vi "Simple TCP - Client.vi"() -> ()   [LabVIEW 2020]
doc: "Demonstrates how to open a connection to an TCP server, read the data being sent, and display the data on a chart. This VI is designed to stop if the TCP connection is terminated."
panel:
  out "data out":string
  in  "Server Closed":string="The server VI closed the connection."
  # "Overview: Demonstrates the use of the TCP functions to connect to a TCP server VI and receive data.\nInstructions:\n1. Ensure Simple TCP - Server.vi is already running.\n2. Run the VI.\n3. Click Stop to stop the VI. Note that if you stop the server VI, this VI will stop automatically."
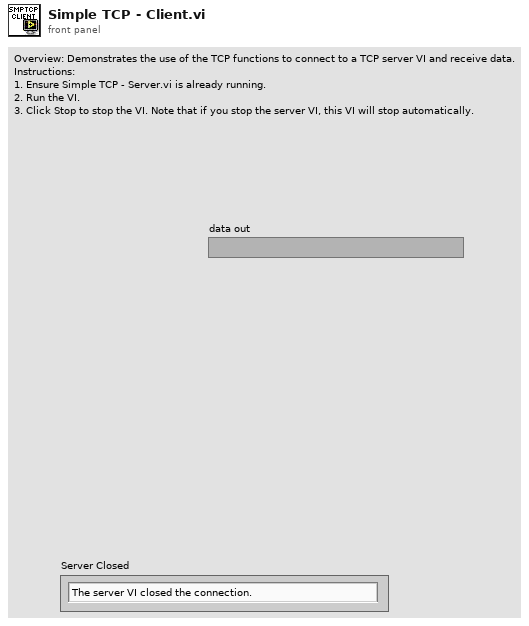
[diagram p1: front panel]
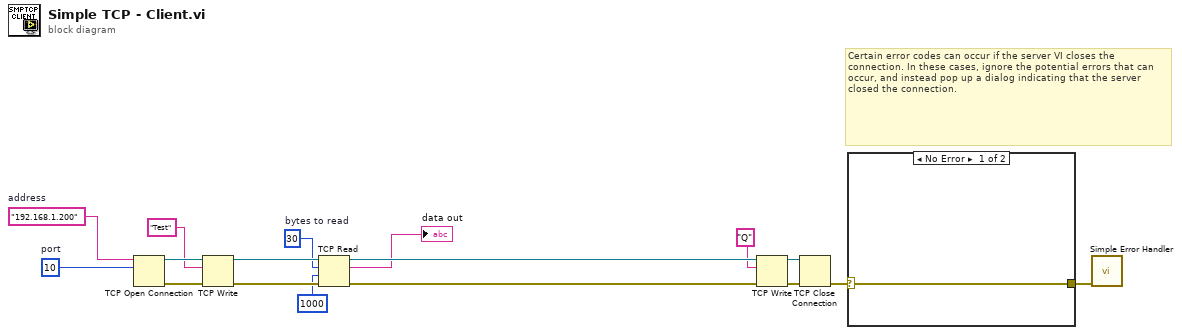
[diagram p0: block diagram]
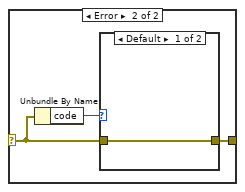
[diagram p2: hidden frame]
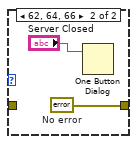
[diagram p3: hidden frame]
diagram:
  w3 = 30  # bytes to read
  w9 = u16 10  # port
  w10 = "192.168.1.200"  # address
  # "Certain error codes can occur if the server VI closes the connection. In these cases, ignore the potential errors that can occur, and instead pop up a dialog indicating that the server closed the connection."
  n1 = TCP Open Connection(address=w10, remote port or service name=w9) -> (connection ID=w8:refnum<k5>, error out=w7:errorcluster)  [unwired: 3 in]
  n2 = TCP Write(connection ID=w8, data in="Test", error in (no error)=w7) -> (connection ID out=w5:refnum<k5>, error out=w6:errorcluster)  [unwired: 1 in, 1 out]
  n3 = TCP Read(connection ID=w5, bytes to read=w3, error in (no error)=w6, 9:1000 ("timeout ms (25000)")) -> (connection ID out=w16:refnum<k5>, data out=→"data out":string, error out=w14:errorcluster)  [unwired: 1 in]
  n4 = TCP Write(connection ID=w16, data in="Q", error in (no error)=w14) -> (connection ID out=w17:refnum<k5>, error out=w15:errorcluster)  [unwired: 2 out]
  n5 = TCP Close Connection(connection ID=w17, error in (no error)=w15) -> (error out=w12:errorcluster)  [unwired: 1 in, 1 out]
  n6 = case shown="No Error" w12 {
    selector: w12 -> [w18 w20]
    tunnel: [w18 w19] -> w11
    frame No Error {
    }
    frame Error {
      n7 = Unbundle By Name(w20) -> ("code"=w21:i32)
      n8 = case shown="Default" w21 {
        tunnel: w20 -> [w22 _]
        tunnel: [w22 w24] -> w19
        frame Default {
        }
        frame 62, 64, 66 {
          w24 = errorcluster {"status"=FALSE, "code"=0, "source"=""}  # No error
          n9 = One Button Dialog(message="Server Closed") -> ()  [unwired: 1 in, 1 out]
        }
      }
    }
  }
  n10 = call <vilib>:"Simple Error Handler.vi"("error in (no error)"=w11) -> ()  [unwired: 4 in, 5 out]
